vi "IncorrectResponse.vi"(8 "error in (no error)":errorcluster, 11 "TrialBasedExperiment in":refnum<class "MatlabExperiment.lvclass">) -> (0 "error out":errorcluster, 3 "TrialBasedExperiment out":refnum<class "MatlabExperiment.lvclass">)   [LabVIEW 2012, in "AcquisitionCoreObjects.lvlib" / "MatlabExperiment.lvclass"]
uses:
  MatlabExperiment.lvclass
  TrialBasedExperimentObject/TrialBasedExperiment.lvclass
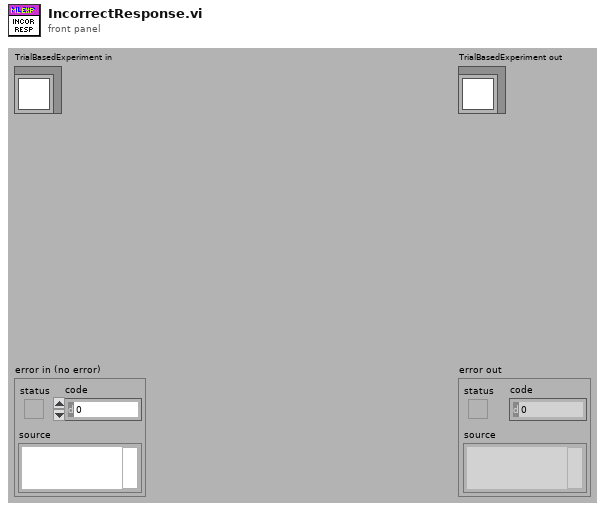
[diagram p1: front panel]
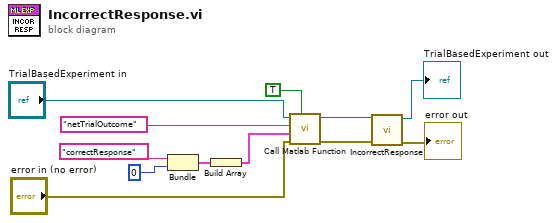
[diagram p0: block diagram]
diagram:
  n1 = Bundle("correctResponse", 0) -> (w10:cluster{string, i32})  [unwired: 1 out]
  n2 = Build Array(w10) -> (w9:cluster{string, i32}[])
  n3 = call-dynamic "Call Matlab Function.vi"("Timestamp"=TRUE, "error in (no error)"="error in (no error)", "Matlab Param Array"=w9, "Function name"="netTrialOutcome", "TrialBasedExperiment in"="TrialBasedExperiment in") -> ("error out"=w4:errorcluster, "TrialBasedExperiment out"=w5:refnum<class "MatlabExperiment.lvclass">)  [unwired: 3 in, 2 out]
  n4 = call-parent "IncorrectResponse.vi"("error in (no error)"=w4, "TrialBasedExperiment in"=w5) -> ("error out"=→"error out":errorcluster, "TrialBasedExperiment out"=→"TrialBasedExperiment out":refnum<class "MatlabExperiment.lvclass">)  [unwired: 8 in]
